vi "Merge Section into Object.vi"(6 "Path to Section (Cluster Name)":string, 7 "error in (no error)":errorcluster, 8 "Section Cluster (or Array of Variants)":variant, 9 "Offset":i32, 10 "JSON Object to merge into":string="{}") -> (0 "error out":errorcluster, 3 "<JSON>":string)   [LabVIEW 2015, in "JSONtext.lvlib"]
doc: "Merges a Section Cluster into JSON Object. A \"Section Cluster\" is defined in analogy to the OpenG Variant Config Library \"Section Cluster\" functions, using a JSON Object, with subObjects representing \"Sections\", instead of INI format.\n\nMerging means that each element of the Section Cluster is inserted into the JSON \"Section\" (Object Item), using the data name of the cluster element. If a Path to the Section is not specified then the data name of the cluster is used. The Section is created if it does not exist.\n\nFor example, Merging the Cluster \"Settings\" with elements A=123 and B=\"test\" into {\"C\":2,\"Settings\":{\"A\"=6,\"D\":9}} would result in:\n{\"C\":2,\"Settings\":{\"A\"=123,\"D\":9,\"B\":\"test\"}}\n\nNote that this merging is not recursive into subClusters."
uses:
  JSONtext.lvlib
  <vilib>/Utility/Data Type/NI_Data Type.lvlib
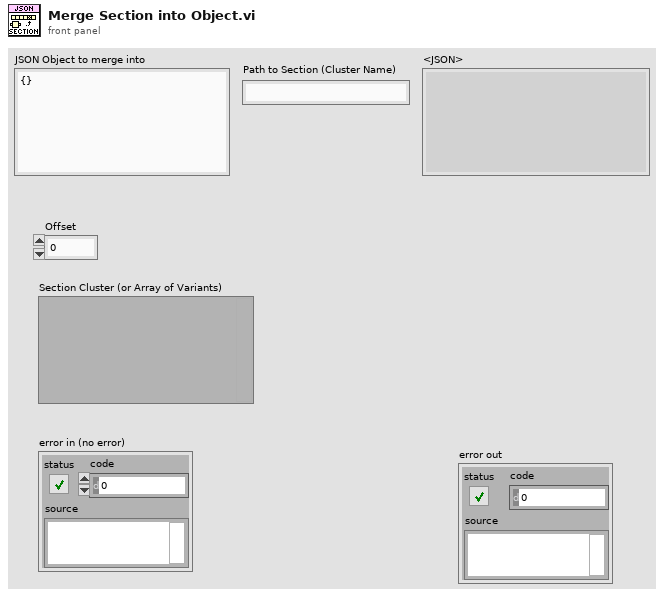
[diagram p1: front panel]
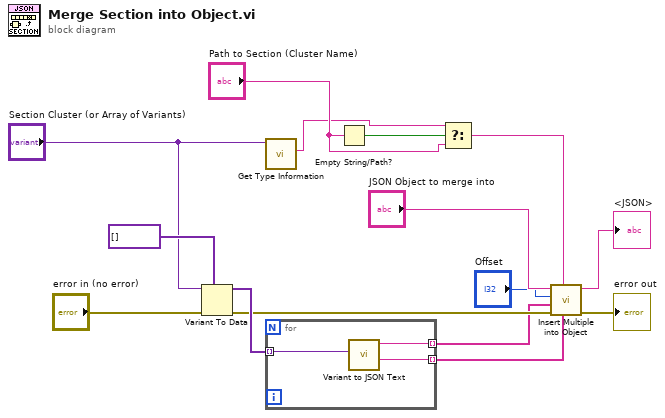
[diagram p0: block diagram]
diagram:
  n1 = Variant To Data(error in="error in (no error)", type=variant[] [], Variant="Section Cluster (or Array of Variants)") -> (data=w10:variant[], error out=w8:errorcluster)
  n2 = call <vilib>:"Get Type Information.vi"("Variant"="Section Cluster (or Array of Variants)") -> ("Name"=w1:string)  [unwired: 6 in, 4 out]
  n3 = for {
    tunnel: w10 -> [w18] mode=indexing
    tunnel: [w17] -> w6 mode=indexing
    tunnel: [w16] -> w7 mode=indexing
    n4 = call "Variant to JSON Text.vi"("Variant"=w18) -> ("Name of data in Variant"=w17:string, "<JSON>"=w16:string)  [unwired: 8 in, 1 out]
  }
  n5 = Empty String/Path?(string/path="Path to Section (Cluster Name)") -> (empty?=w4:bool)
  n6 = Select(t=w1, s=w4, f="Path to Section (Cluster Name)") -> (s? t:f=w3:string)
  n7 = call "Insert Multiple into Object.vi"("Item Names"=w6, "Object Path"=w3, "error in (no error)"=w8, "JSON to Insert"=w7, "Object Offset"="Offset", "JSON in"="JSON Object to merge into") -> ("error out"=→"error out":errorcluster, "<JSON>"=→"<JSON>":string)  [unwired: 3 in]
